vi "Close.vi"(8 "error in (no error)":errorcluster, 11 "navX - SPI in":refnum<class "navX - SPI.lvclass">) -> (0 "error out":errorcluster, 1 "Timed out?":bool, 3 "navX - SPI out":refnum<class "navX - SPI.lvclass">)   [LabVIEW 2015, in "navX Library v3.lvlib" / "navX - SPI.lvclass"]
uses:
  navX - SPI.lvclass
  navX - SPI.lvclass/navX - SPI.ctl
  navX - Interface/navX - Interface.lvclass
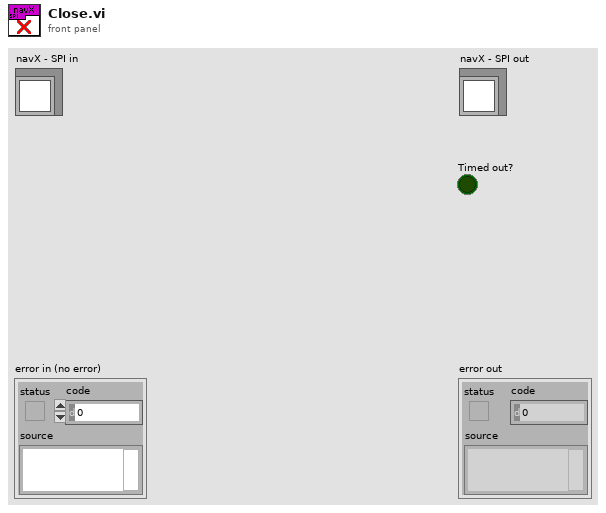
[diagram p1: front panel]
types:
  T1 = typedef "WPI_SPIDevRef.ctl" = cluster{"DevStatus":errorcluster, "Handle":i32, "SPI Bus":T2}
  T2 = typedef "spi_bus.ctl" = enum16{"SPI On-Board, CS0", "SPI On-Board, CS1", "SPI On-Board, CS2", "SPI On-Board, CS3", "SPI MXP", "Invalid"}
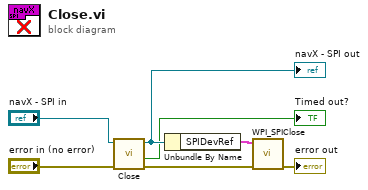
[diagram p0: block diagram]
diagram:
  n1 = call-parent "Close.vi"("error in (no error)"="error in (no error)", "navX - Base in"="navX - SPI in") -> ("error out"=w7:errorcluster, "Timed out?"=→"Timed out?":bool, "navX - Base out"=w3:refnum<class "navX - SPI.lvclass">)  [unwired: 7 in]
  "navX - SPI out" <- w3
  n2 = Unbundle By Name(w3) -> ("SPIDevRef"=w2:T1)
  n3 = call <vilib>:"WPI_SPIClose.vi"("error in (no error)"=w7, "SPIDevRef"=w2) -> ("error out"=→"error out":errorcluster)  [unwired: 9 in]
